vi "CompoundShape.vi"(8 "error in (no error)":errorcluster, 10 "id":i32, 11 "CompoundShape in":refnum<class "CompoundShape.lvclass">) -> (0 "error out":errorcluster, 3 "CompoundShape out":refnum<class "CompoundShape.lvclass">)   [LabVIEW 2017, in "CompoundShape.lvclass"]
uses:
  CompoundShape.lvclass
  CompoundShape.lvclass/CompoundShape.ctl
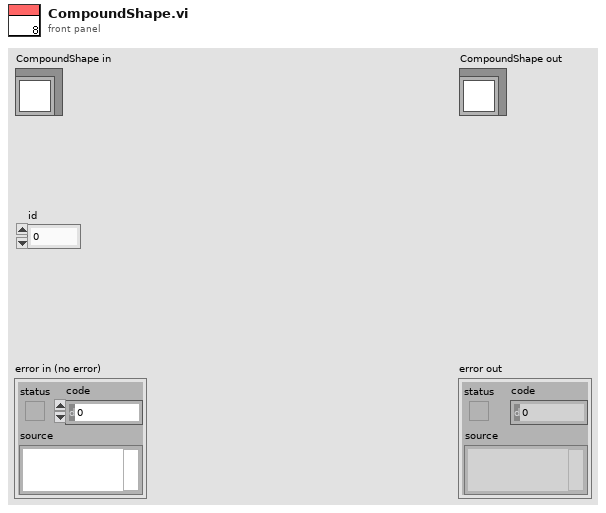
[diagram p1: front panel]
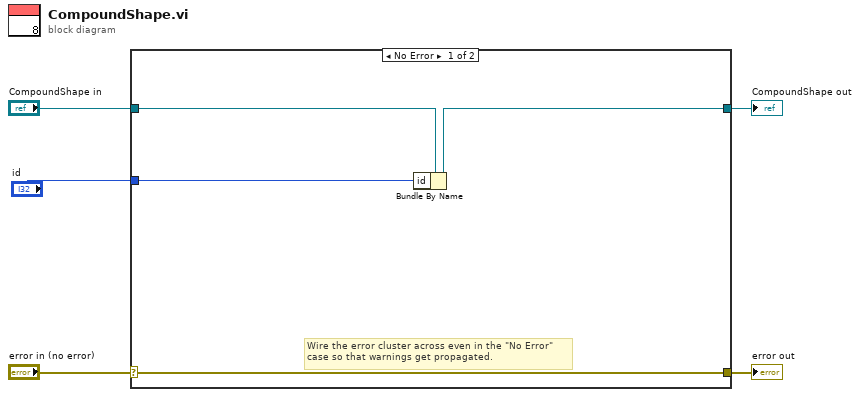
[diagram p0: block diagram]
diagram:
  n1 = case shown="No Error" "error in (no error)" {
    selector: "error in (no error)" -> [w8 w11]
    tunnel: [w8 w11] -> w4
    tunnel: [w7 w10] -> w2
    tunnel: "CompoundShape in" -> [w9 w10]
    tunnel: "id" -> [w6 _]
    frame No Error {
      # "Wire the error cluster across even in the \"No Error\"\ncase so that warnings get propagated."
      n2 = Bundle By Name(cluster=w9, "id"=w6) -> (w7:refnum<class "CompoundShape.lvclass">)
    }
    frame Error {
    }
  }
  "error out" <- w4
  "CompoundShape out" <- w2
